vi "mqttClient_Viewer.vi"() -> ()   [LabVIEW 2019]
uses:
  <vilib>/LabVIEW Open Source Project/OpenSerializer JKI JSON/Serializer.JSON.lvclass
  C:/Program Files (x86)/National Instruments/LabVIEW 2019/vi.lib/LabVIEW Open Source Project/OpenSerializer/Serializer/Serializer.lvclass
  state -- cluster.ctl
  <vilib>/LabVIEW Open Source Project/MQTT Connection/MQTT_Base/Base Class/MQTT_Base.lvclass/MQTT_Base.ctl
  <vilib>/LabVIEW Open Source Project/MQTT Client/Client class/Client.lvclass/Client.ctl
  target -- cluster.ctl
  <vilib>/LabVIEW Open Source Project/MQTT Control Packets/Control Packets/ControlPacket/QualityOfService -- enum.ctl
  <vilib>/LabVIEW Open Source Project/MQTT Control Packets/Control Packets/ControlPacket/ControlPacket.lvclass/ControlPacket.ctl
  <vilib>/LabVIEW Open Source Project/MQTT Control Packets/Control Packets/CONNECT/ConnectFlags -- cluster.ctl
  <vilib>/LabVIEW Open Source Project/MQTT TCP Connection/MQTT_TCP/Connection/TCPConnection.lvclass
  C:/Program Files (x86)/National Instruments/LabVIEW 2019/vi.lib/LabVIEW Open Source Project/MQTT Connection/MQTT_Connection/Connection/Connection.lvclass
  <vilib>/LabVIEW Open Source Project/MQTT Client/Client class/Client.lvclass
  C:/Program Files (x86)/National Instruments/LabVIEW 2019/vi.lib/LabVIEW Open Source Project/MQTT Connection/MQTT_Base/Base Class/MQTT_Base.lvclass
  <vilib>/LabVIEW Open Source Project/OpenSerializer/Serializer.FlattenedString/Serializer.FlattenedString.lvclass
  <vilib>/LabVIEW Open Source Project/MQTT Control Packets/Control Packets/PUBLISH/PUBLISH.lvclass
  C:/Program Files (x86)/National Instruments/LabVIEW 2019/vi.lib/LabVIEW Open Source Project/MQTT Control Packets/Control Packets/ControlPacket/ControlPacket.lvclass
  <vilib>/LabVIEW Open Source Project/OpenSerializer/Serializer/Serializer.lvclass
  <vilib>/LabVIEW Open Source Project/MQTT Connection/MQTT_Base/Base Class/MQTT_Base.lvclass
  <vilib>/LabVIEW Open Source Project/MQTT Control Packets/Control Packets/CONNECT/CONNECT.lvclass
  <vilib>/LabVIEW Open Source Project/MQTT Control Packets/Control Packets/ControlPacket/ControlPacket.lvclass
panel:
  out "Incoming Messages":string
  in  "Connection":bool
  out "last error":errorcluster
  in  "setpoint":dbl format="%.1g"
  in  "enabled":bool
  out "Waveform Chart":cluster{"setpoint":dbl, "measured":dbl}(graph)
  # "Native LabVIEW MQTT Client (View)"
  # "G Open Source Project for LabVIEW\nhttps://github.com/LabVIEW-Open-Source/MQTT-Client"
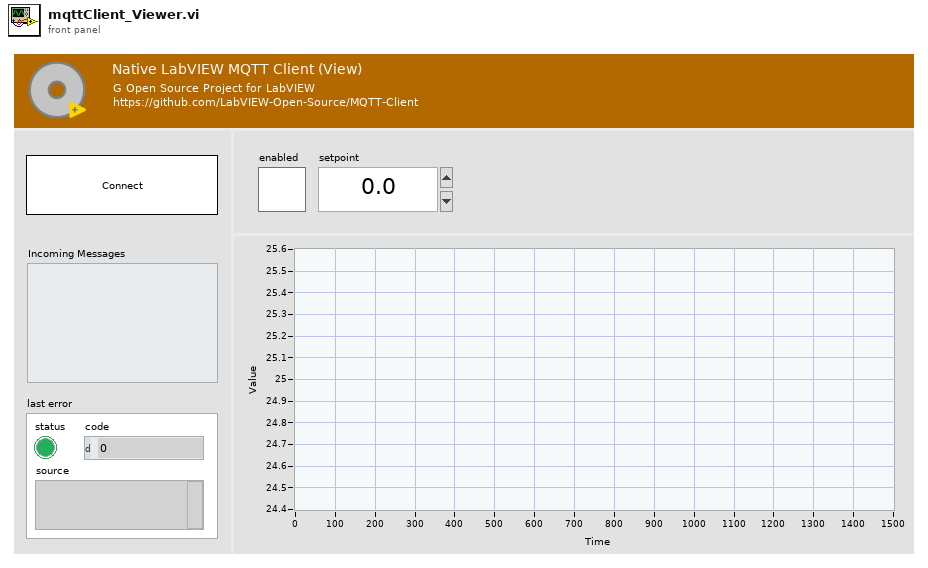
[diagram p1: front panel]
types:
  T1 = typedef "state -- cluster.ctl" = cluster{"enabled":bool, "setpoint":dbl, "measured":dbl}
  T2 = typedef "MQTT Client.lvlib/Client.lvclass/Public Events -- cluster.ctl" = cluster{"Connection Status":refnum<user-event>, "Connected":refnum<user-event>, "Application Message":refnum<user-event>}
  T3 = typedef "MQTT Base.lvlib/MQTT_Base.lvclass/Public Events -- cluster.ctl" = cluster{"Stop Event":refnum<user-event>, "Error Event":refnum<user-event>, "Inbound Message":refnum<user-event>}
  T4 = typedef "MQTT_Control_Packets.lvlib/ControlPacket.lvclass/QualityOfService -- enum.ctl" = enum16{"0 (At Most Once)", "1 (At Least Once)", "2 (Exactly Once)"}
  T5 = typedef "MQTT_Control_Packets.lvlib/CONNECT.lvclass/ConnectFlags -- cluster.ctl" = cluster{"Reserved":bool, "Clean Session":bool, "Will Flag":bool, "Will QoS 1":bool, "Will QoS 2":bool, "Will Retain":bool, "Password Flag":bool, "User Name Flag":bool}
  T6 = typedef "target -- cluster.ctl" = cluster{"enabled":bool, "setpoint":dbl, "responseURI":string}
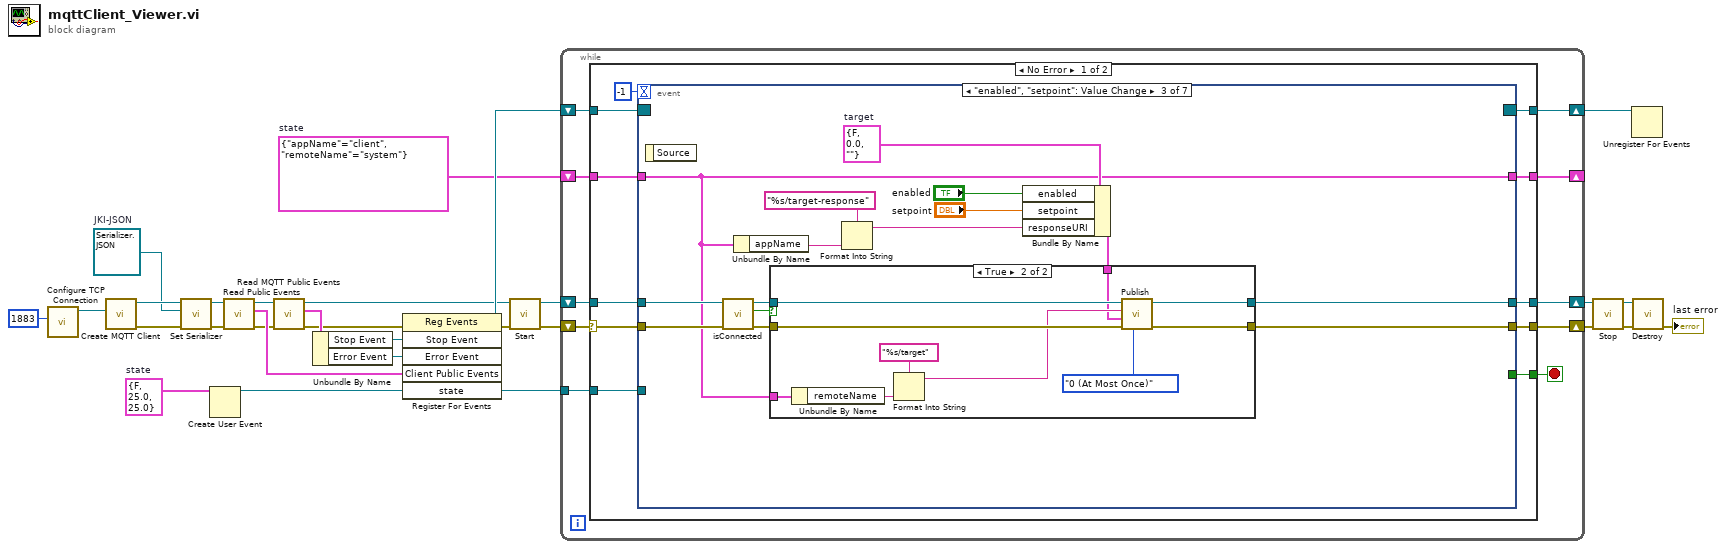
[diagram p0: block diagram]
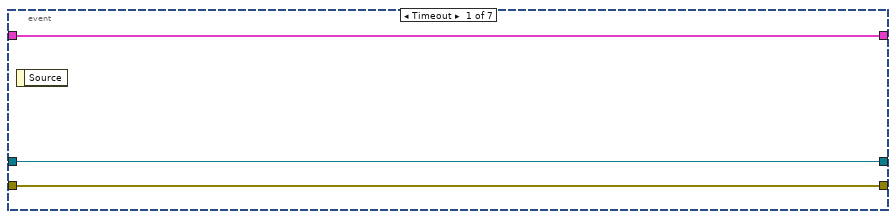
[diagram p2: hidden frame]
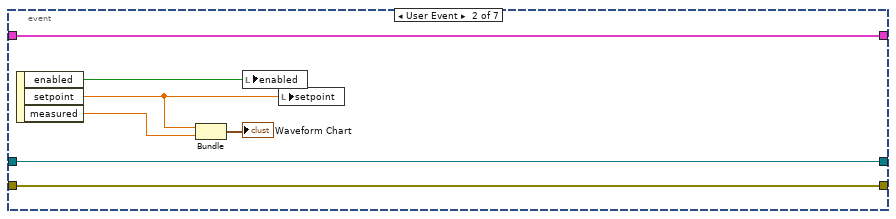
[diagram p3: hidden frame]
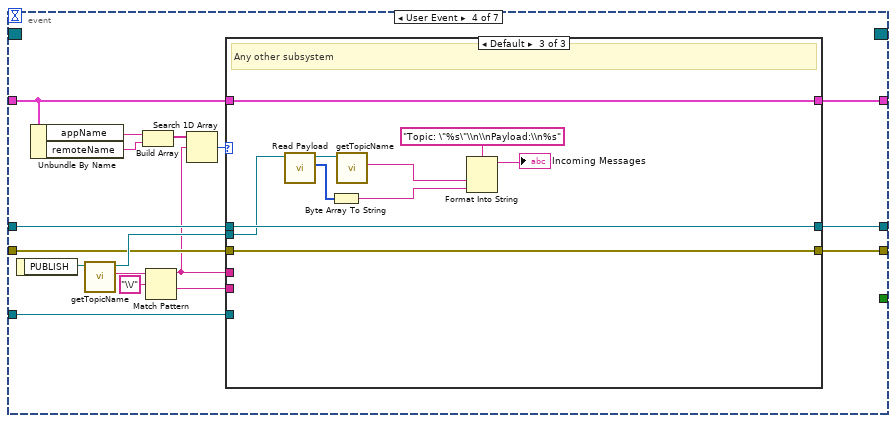
[diagram p5: hidden frame]
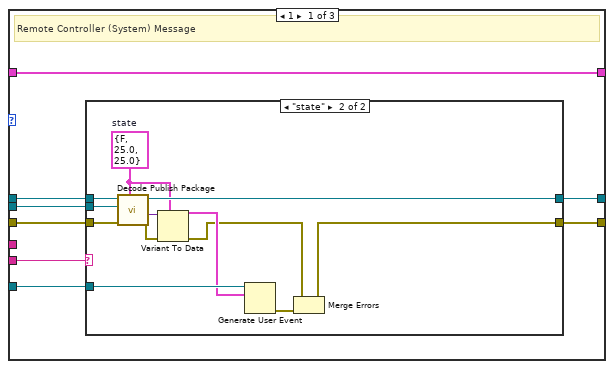
[diagram p6: hidden frame]
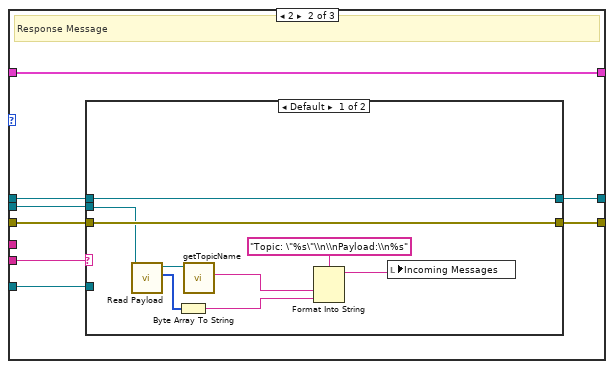
[diagram p8: hidden frame]
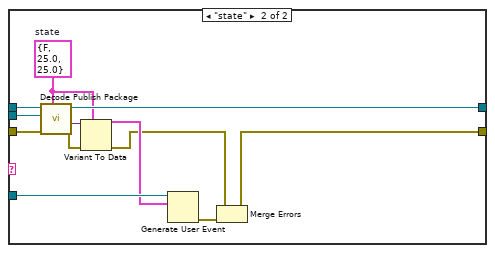
[diagram p9: hidden frame]
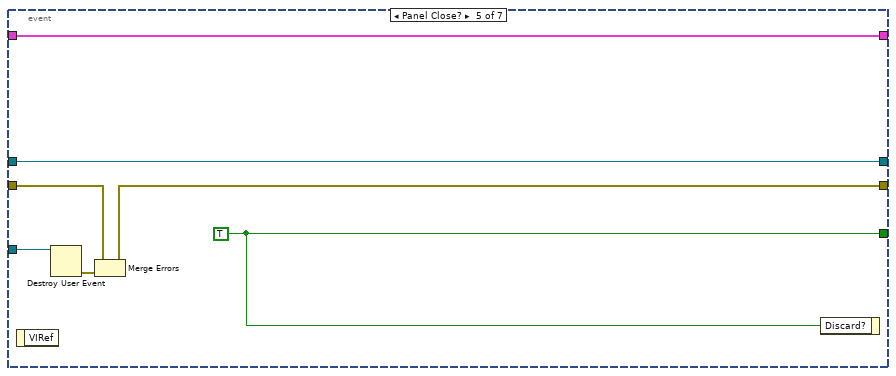
[diagram p10: hidden frame]
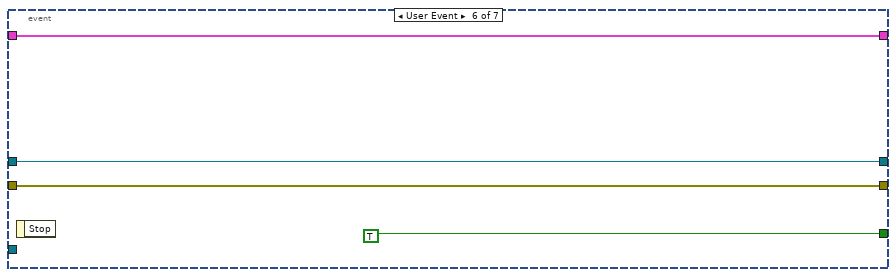
[diagram p11: hidden frame]
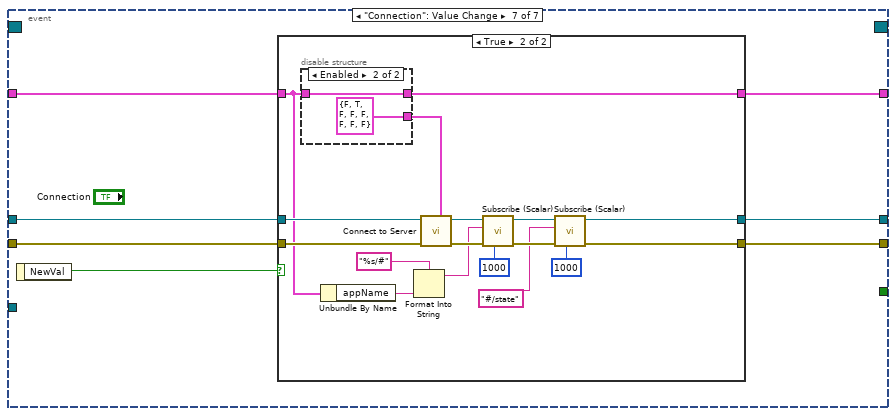
[diagram p12: hidden frame]
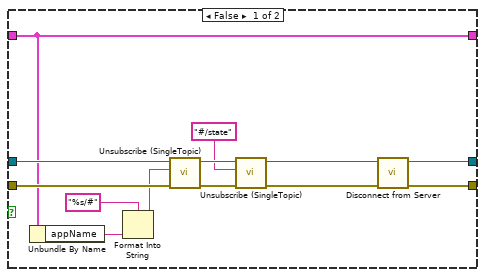
[diagram p13: hidden frame]
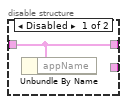
[diagram p14: hidden frame]
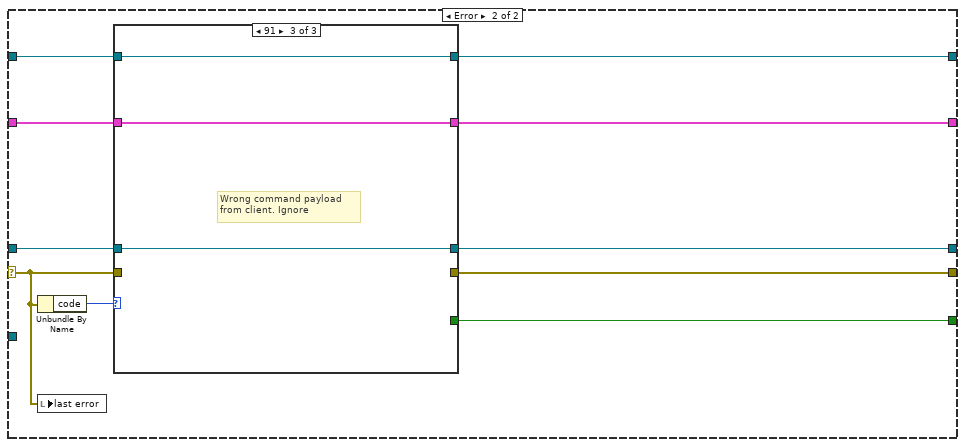
[diagram p15: hidden frame]
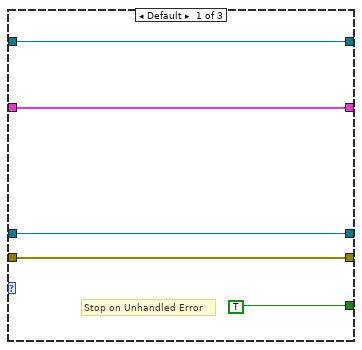
[diagram p16: hidden frame]
diagram:
  w2 = T1 {"enabled"=FALSE, "setpoint"=25.0, "measured"=25.0}  # state
  w3 = cluster{"appName":string, "remoteName":string} {"appName"="client", "remoteName"="system"}  # state
  w6 = refnum<class "Serializer.JSON.lvclass"> refnum  # JKI-JSON
  n1 = call <vilib>:"Configure TCP Connection.vi"("remote port (80)"=u16 1883) -> ("TCPConnection"=w11:refnum<class "TCPConnection.lvclass">)  [unwired: 9 in, 1 out]
  n2 = call <vilib>:"Create MQTT Client.vi"("Connection Configuration"=w11) -> ("error out"=w8:errorcluster, "Client out"=w10:refnum<class "Client.lvclass">)  [unwired: 9 in]
  n3 = call <vilib>:"Set Serializer.vi"("error in (no error)"=w8, "Serializer (default: Flattened String)"=w6, "MQTT_Base"=w10) -> ("error out"=w7:errorcluster, "MQTT_Base out"=w9:refnum<class "Client.lvclass">)  [unwired: 7 in]
  n4 = Create User Event(user event datatype=w2) -> (user event=w1:refnum<user-event>)  [unwired: 1 in, 1 out]
  n5 = call <vilib>:"Read Public Events.vi"("error in (no error)"=w7, "Client in"=w9) -> ("error out"=w13:errorcluster, "Client Public Events"=w15:T2, "Client out"=w12:refnum<class "Client.lvclass">)  [unwired: 7 in]
  n6 = call <vilib>:"Read MQTT Public Events.vi"("error in (no error)"=w13, "MQTT_Base in"=w12) -> ("error out"=w14:errorcluster, "MQTT Public Events"=w22:T3, "MQTT_Base out"=w17:refnum<class "Client.lvclass">)  [unwired: 7 in]
  n7 = Unbundle By Name(w22) -> ("Stop Event"=w20:refnum<user-event>, "Error Event"=w21:refnum<user-event>)
  n8 = register-events(error in=w14, w20, w21, w15, w1) -> (reference out=w18:refnum<event-registration>, error out=w16:errorcluster)  [unwired: 1 in]
  n9 = call <vilib>:"Start.vi"("error in (no error)"=w16, "MQTT_Base in"=w17) -> ("error out"=w4:errorcluster, "MQTT_Base out"=w5:refnum<class "Client.lvclass">)  [unwired: 7 in, 1 out]
  n10 = while {
    shift-right: [w37] -> w19
    shift-left: w18 -> [w38]
    shift-right: [w34] -> w24
    shift-left: w5 -> [w35]
    shift-right: [w36] -> w26
    shift-left: w4 -> [w32]
    shift-right: [w30] -> _
    shift-left: w3 -> [w31]
    tunnel: w1 -> [w29]
    stop <- w33 stop-if-true
    n11 = case shown="No Error" w32 {
      selector: w32 -> [w42 w219]
      tunnel: w38 -> [w49 w218]
      tunnel: [w48 w217] -> w37
      tunnel: [w47 w222] -> w36
      tunnel: w35 -> [w45 w223]
      tunnel: [w44 w225] -> w34
      tunnel: [w43 w221] -> w33
      tunnel: w31 -> [w41 w220]
      tunnel: [w40 w216] -> w30
      tunnel: w29 -> [w39 _]
      frame No Error {
        n12 = event shown="[2] \"enabled\", \"setpoint\": Value Change" {
          selector: w49 -> [_ _ _ _ _ _ _]
          dyn-events: [_ _ _ _ _ _ _] -> w48
          timeout: -1 -> [_ _ _ _ _ _ _]
          tunnel: w42 -> [w50 w57 w70 w100 w165 w175 w178]
          tunnel: [w50 w57 w65 w98 w166 w175 w179] -> w47
          tunnel: [_ _ _ _ w171 TRUE _] -> w43
          tunnel: w45 -> [w51 w58 w71 w101 w170 w173 w182]
          tunnel: [w51 w58 w66 w99 w170 w173 w180] -> w44
          tunnel: w41 -> [w52 w59 w62 w93 w169 w172 w176]
          tunnel: [w52 w59 w62 w97 w169 w172 w177] -> w40
          tunnel: w39 -> [_ _ _ w92 w168 _ _]
          event Timeout {
            n13 = event-data() -> ()  [unwired: 1 in, 1 out]
          }
          event User Event {
            n14 = event-data() -> ("enabled"=w55:bool, "setpoint"=w53:dbl, "measured"=w54:dbl)  [unwired: 1 in]
            n15 = Bundle("setpoint"=w53, "measured"=w54) -> (→"Waveform Chart":cluster{"setpoint":dbl, "measured":dbl})  [unwired: 1 in]
            n16 = local write "enabled"(w55) -> ()
            n17 = local write "setpoint"(w53) -> ()
          }
          event "enabled", "setpoint": Value Change {
            w64 = T6 {"enabled"=FALSE, "setpoint"=0.0, "responseURI"=""}  # target
            n18 = event-data() -> ()  [unwired: 1 in, 1 out]
            n19 = call <vilib>:"isConnected.vi"("error in (no error)"=w70, "Client in"=w71) -> ("error out"=w74:errorcluster, "connected"=w72:bool, "Client out"=w73:refnum<class "Client.lvclass">)  [unwired: 7 in]
            n20 = Unbundle By Name(w62) -> ("appName"=w61:string)
            n21 = Format Into String(format string="%s/target-response" ("Topic Name (empty: Payload name)"), w61) -> (resulting string=w63:string)  [unwired: 2 in, 1 out]
            n22 = Bundle By Name(cluster=w64, "enabled"="enabled", "setpoint"="setpoint", "responseURI"=w63) -> (w67:T6)
            n23 = case shown="True" w72 {
              tunnel: [w76 w85] -> w66
              tunnel: [w75 w83] -> w65
              tunnel: w73 -> [w76 w86]
              tunnel: w74 -> [w75 w84]
              tunnel: w62 -> [_ w78]
              tunnel: w67 -> [_ w77]
              frame False {
              }
              frame True {
                n24 = Unbundle By Name(w78) -> ("remoteName"=w81:string)
                n25 = Format Into String(format string="%s/target" ("Topic Name (empty: Payload name)"), w81) -> (resulting string=w79:string)  [unwired: 2 in, 1 out]
                n26 = call <vilib>:"Publish.vi"("QoS"=QualityOfService_--_enum."0 (At Most Once)", "error in (no error)"=w84, "Payload"=w77, "Topic Name (empty: Payload name)"=w79, "Client in"=w86) -> ("error out"=w83:errorcluster, "Client out"=w85:refnum<class "Client.lvclass">)  [unwired: 4 in, 1 out]
              }
            }
          }
          event User Event {
            n27 = event-data() -> ("PUBLISH"=w103:refnum<class "PUBLISH.lvclass">)  [unwired: 1 in]
            n28 = Unbundle By Name(w93) -> ("appName"=w91:string, "remoteName"=w90:string)
            n29 = call <vilib>:"getTopicName.vi"("PUBLISH in"=w103) -> ("Topic"=w95:string, "PUBLISH out"=w102:refnum<class "PUBLISH.lvclass">)  [unwired: 8 in, 1 out]
            n30 = Build Array(w91, w90) -> (w89:string[])
            n31 = Match Pattern(string=w95, regular expression="\\/") -> (before substring=w88:string, after substring=w94:string)  [unwired: 1 in, 2 out]
            n32 = Search 1D Array(1D array=w89, element=w88) -> (index of element=w87:i32)  [unwired: 1 in]
            n33 = case shown="Default" w87 {
              tunnel: w102 -> [w108 w130 w155]
              tunnel: w101 -> [w110 w132 w163]
              tunnel: w100 -> [w109 w131 w162]
              tunnel: [w107 w129 w163] -> w99
              tunnel: [w106 w128 w162] -> w98
              tunnel: w93 -> [w111 w133 w164]
              tunnel: [w111 w133 w164] -> w97
              tunnel: w94 -> [w105 w127 _]
              tunnel: w88 -> [_ _ _]
              tunnel: w92 -> [w104 w126 _]
              frame 1 {
                # "Remote Controller (System) Message"
                n34 = case shown="\"state\"" w105 {
                  tunnel: w110 -> [w113 w125]
                  tunnel: w109 -> [w112 w124]
                  tunnel: w108 -> [_ w123]
                  tunnel: [w113 w122] -> w107
                  tunnel: [w112 w114] -> w106
                  tunnel: w104 -> [_ w118]
                  frame Default {
                  }
                  frame "state" {
                    w119 = T1 {"enabled"=FALSE, "setpoint"=25.0, "measured"=25.0}  # state
                    n35 = call <vilib>:"Decode Publish Package.vi"("Type"=w119, "error in (no error)"=w124, "PUBLISH"=w123, "MQTT_Base in"=w125) -> ("error out"=w120:errorcluster, "Payload"=w121:variant, "MQTT_Base out"=w122:refnum<class "Client.lvclass">)  [unwired: 4 in, 1 out]
                    n36 = Variant To Data(error in=w120, type=w119, Variant=w121) -> (data=w117:T1, error out=w115:errorcluster)
                    n37 = Generate User Event(user event=w118, event data cluster=w117) -> (error out=w116:errorcluster)  [unwired: 2 in, 1 out]
                    n38 = Merge Errors(w115, w116) -> (w114:errorcluster)
                  }
                }
              }
              frame 2 {
                # "Response Message"
                n39 = case shown="Default" w127 {
                  tunnel: w132 -> [w142 w154]
                  tunnel: w131 -> [w141 w153]
                  tunnel: w130 -> [w135 w152]
                  tunnel: [w142 w151] -> w129
                  tunnel: [w141 w143] -> w128
                  tunnel: w126 -> [_ w147]
                  frame Default {
                    n40 = call <vilib>:"Read Payload.vi"("ControlPacket in"=w135) -> ("Payload"=w140:u8[], "ControlPacket out"=w139:refnum<class "PUBLISH.lvclass">)  [unwired: 9 in]
                    n41 = Byte Array To String(unsigned byte array=w140) -> (string=w138:string)
                    n42 = call <vilib>:"getTopicName.vi"("PUBLISH in"=w139) -> ("Topic"=w137:string)  [unwired: 8 in, 2 out]
                    n43 = Format Into String(format string="Topic: \"%s\"\\n\\nPayload:\\n%s", w137, w138) -> (resulting string=w134:string)  [unwired: 2 in, 1 out]
                    n44 = local write "Incoming Messages"(w134) -> ()
                  }
                  frame "state" {
                    w148 = T1 {"enabled"=FALSE, "setpoint"=25.0, "measured"=25.0}  # state
                    n45 = call <vilib>:"Decode Publish Package.vi"("Type"=w148, "error in (no error)"=w153, "PUBLISH"=w152, "MQTT_Base in"=w154) -> ("error out"=w149:errorcluster, "Payload"=w150:variant, "MQTT_Base out"=w151:refnum<class "Client.lvclass">)  [unwired: 4 in, 1 out]
                    n46 = Variant To Data(error in=w149, type=w148, Variant=w150) -> (data=w146:T1, error out=w144:errorcluster)
                    n47 = Generate User Event(user event=w147, event data cluster=w146) -> (error out=w145:errorcluster)  [unwired: 2 in, 1 out]
                    n48 = Merge Errors(w144, w145) -> (w143:errorcluster)
                  }
                }
              }
              frame Default {
                # "Any other subsystem"
                n49 = call <vilib>:"Read Payload.vi"("ControlPacket in"=w155) -> ("Payload"=w161:u8[], "ControlPacket out"=w160:refnum<class "PUBLISH.lvclass">)  [unwired: 9 in]
                n50 = Byte Array To String(unsigned byte array=w161) -> (string=w158:string)
                n51 = call <vilib>:"getTopicName.vi"("PUBLISH in"=w160) -> ("Topic"=w157:string)  [unwired: 8 in, 2 out]
                n52 = Format Into String(format string="Topic: \"%s\"\\n\\nPayload:\\n%s", w157, w158) -> (resulting string=→"Incoming Messages":string)  [unwired: 2 in, 1 out]
              }
            }
          }
          event Panel Close? {
            w171 = TRUE
            n53 = event-data() -> ()  [unwired: 1 in, 1 out]
            n54 = Destroy User Event(user event=w168) -> (error out=w167:errorcluster)  [unwired: 1 in]
            n55 = Merge Errors(w165, w167) -> (w166:errorcluster)
            n56 = event-data("Discard?"=w171) -> ()  [unwired: 1 in, 1 out]
          }
          event User Event {
            n57 = event-data() -> ()  [unwired: 1 in, 1 out]
          }
          event "Connection": Value Change {
            n58 = event-data() -> ("NewVal"=w181:bool)  [unwired: 1 in]
            n59 = case shown="True" w181 {
              tunnel: w182 -> [w193 w212]
              tunnel: [w195 w198] -> w180
              tunnel: [w194 w197] -> w179
              tunnel: w178 -> [w192 w211]
              tunnel: [w189 w210] -> w177
              tunnel: w176 -> [w189 w204]
              frame False {
                n60 = Unbundle By Name(w189) -> ("appName"=w191:string)
                n61 = Format Into String(format string="%s/#" ("Topic Name (empty: Payload name)"), w191) -> (resulting string=w188:string)  [unwired: 2 in, 1 out]
                n62 = call <vilib>:"Unsubscribe (SingleTopic).vi"("error in (no error)"=w192, "Topic Filter"=w188, "MQTT_Base in"=w193) -> ("error out"=w187:errorcluster, "MQTT_Base out"=w186:refnum<class "Client.lvclass">)  [unwired: 6 in, 1 out]
                n63 = call <vilib>:"Unsubscribe (SingleTopic).vi"("error in (no error)"=w187, "Topic Filter"="#/state" ("Topic Name (empty: Payload name)"), "MQTT_Base in"=w186) -> ("error out"=w184:errorcluster, "MQTT_Base out"=w185:refnum<class "Client.lvclass">)  [unwired: 6 in, 1 out]
                n64 = call <vilib>:"Disconnect from Server.vi"("error in (no error)"=w184, "Client in"=w185) -> ("error out"=w194:errorcluster, "Client out"=w195:refnum<class "Client.lvclass">)  [unwired: 7 in, 1 out]
              }
              frame True {
                n65 = disable-structure shown="Enabled" {
                  disable-tunnel: w204 -> [w213 w215]
                  disable-tunnel: [w213 w215] -> w210
                  disable-tunnel: [_ T5 {"Reserved"=FALSE, "Clean Session"=TRUE, "Will Flag"=FALSE, "Will QoS 1"=FALSE, "Will QoS 2"=FALSE, "Will Retain"=FALSE, "Password Flag"=FALSE, "User Name Flag"=FALSE} ("Connect Flags")] -> w209
                  frame Disabled {
                    n66 = Unbundle By Name(w213) -> ()  [unwired: 1 out]
                  }
                  frame Enabled {
                  }
                }
                n67 = Unbundle By Name(w204) -> ("appName"=w205:string)
                n68 = Format Into String(format string="%s/#" ("Topic Name (empty: Payload name)"), w205) -> (resulting string=w202:string)  [unwired: 2 in, 1 out]
                n69 = call <vilib>:"Connect to Server.vi"("Connect Flags"=w209, "error in (no error)"=w211, "Client in"=w212) -> ("error out"=w206:errorcluster, "Client out"=w207:refnum<class "Client.lvclass">)  [unwired: 5 in, 2 out]
                n70 = call <vilib>:"Subscribe (Scalar).vi"("timeout (1000ms)"=1000 ("timeout (100ms)"), "error in (no error)"=w206, "Topic Filter"=w202, "Client in"=w207) -> ("error out"=w199:errorcluster, "Client out"=w200:refnum<class "Client.lvclass">)  [unwired: 5 in, 1 out]
                n71 = call <vilib>:"Subscribe (Scalar).vi"("timeout (1000ms)"=1000 ("timeout (100ms)"), "error in (no error)"=w199, "Topic Filter"="#/state" ("Topic Name (empty: Payload name)"), "Client in"=w200) -> ("error out"=w197:errorcluster, "Client out"=w198:refnum<class "Client.lvclass">)  [unwired: 5 in, 1 out]
              }
            }
          }
        }
      }
      frame Error {
        n72 = Unbundle By Name(w219) -> ("code"=w224:i32)
        n73 = local write "last error"(w219) -> ()
        n74 = case shown="91" w224 {
          tunnel: w223 -> [w230 w233 w236]
          tunnel: [w230 w233 w236] -> w225
          tunnel: w219 -> [w229 _ _]
          tunnel: [w229 _ _] -> w222
          tunnel: [TRUE _ _] -> w221
          tunnel: w220 -> [w226 w231 w234]
          tunnel: w218 -> [w227 w232 w235]
          tunnel: [w227 w232 w235] -> w217
          tunnel: [w226 w231 w234] -> w216
          frame Default {
            # "Stop on Unhandled Error"
          }
          frame 56, 66 {
            # "Disconnected"
          }
          frame 91 {
            # "Wrong command payload\nfrom client. Ignore"
          }
        }
      }
    }
  }
  n75 = call <vilib>:"Stop.vi"("error in (no error)"=w26, "MQTT_Base in"=w24) -> ("error out"=w25:errorcluster, "MQTT_Base out"=w23:refnum<class "Client.lvclass">)  [unwired: 7 in, 1 out]
  n76 = Unregister For Events(event registration refnum=w19) -> ()  [unwired: 1 in, 1 out]
  n77 = call <vilib>:"Destroy.vi"("error in (no error)"=w25, "MQTT_Base in"=w23) -> ("error out"=→"last error":errorcluster)  [unwired: 8 in, 1 out]
